vi "4110_Volt _Chan Config Dialog_RTM.vi"(8 "error in (no error)":errorcluster, 11 "CD PTR":T1 format="%.0x") -> (0 "error out":errorcluster, 1 "Channels to Add":u16[](array[numeric]), 2 "Current Limit (out)":dbl, 3 "Initial Voltage Value (out)":dbl, 5 "Cancel (out)":bool)   [LabVIEW 2018, in "NI PXI-4110 Programmable Power Supply Custom Device.lvlib"]
uses:
  NI PXI-4110 Programmable Power Supply Custom Device.lvlib
  <vilib>/NI Veristand/Custom Device API/Custom Device Item Ref.ctl
  Power_Supply_In_Use.ctl
  4110_Global.vi
  <vilib>/NI Veristand/Custom Device API/Get Item Property (U16).vi
  <vilib>/NI Veristand/Custom Device API/Get Item Property (Boolean).vi
  <vilib>/NI VeriStand/Custom Device API/Custom Device API.lvlib
panel:
  in  "Channel(s) to add":T2
  in  "Cancel":bool
  in  "OK Button":bool
  in  "Current Limit":dbl format="%.4f"
  in  "Initial Voltage Value":dbl
  # "Voltage Channels"
  # "Note: Channel 2 current\nvalues will be converted\nto negative values\nappropriately."
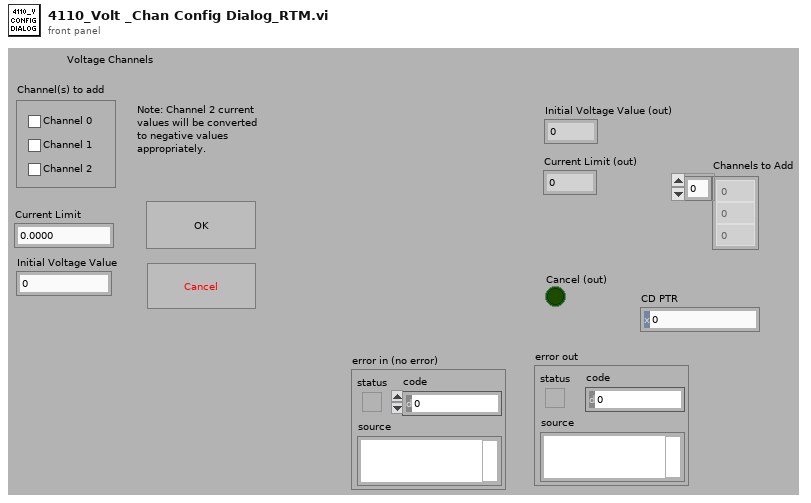
[diagram p1: front panel]
types:
  T1 = typedef "Custom Device API.lvlib/Custom Device Item Ref.ctl" = u64
  T2 = cluster{"Channel 0":bool, "Channel 1":bool, "Channel 2":bool}
  T3 = enum8{"Enabled", "Disabled", "Disabled and Grayed Out"}
  T4 = typedef "NI PXI-4110 Programmable Power Supply Custom Device.lvlib/Power_Supply_In_Use.ctl" = enum16{"PXIe-4112", "PXI-4110"}
  T5 = cluster{"V_min":dbl, "V_max":dbl, "I_min":dbl, "I_max":dbl}
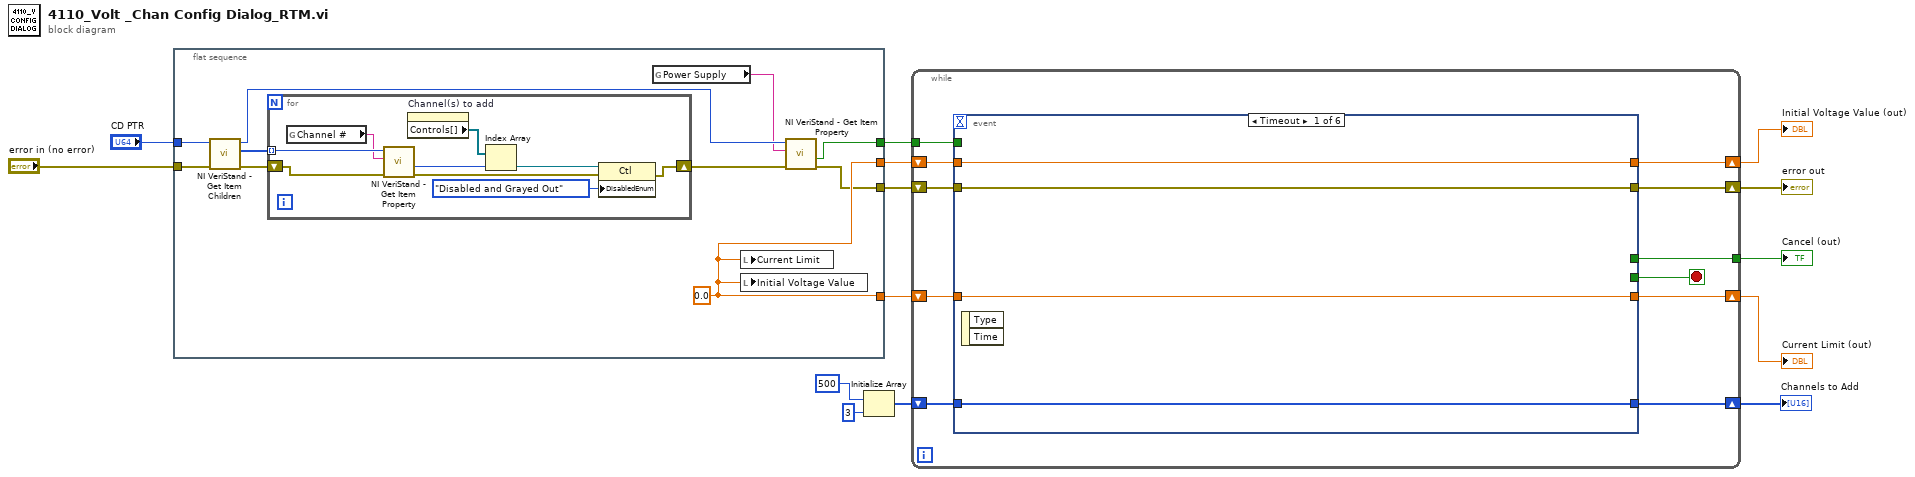
[diagram p0: block diagram]
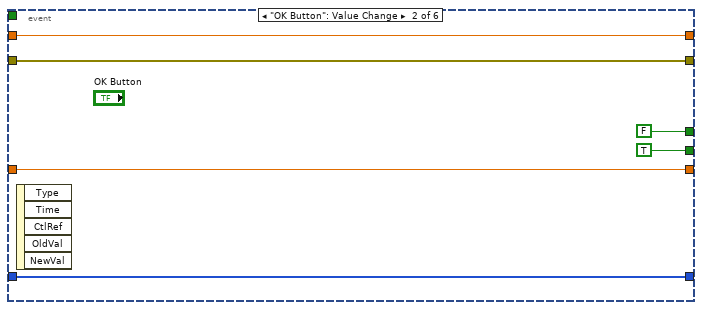
[diagram p2: hidden frame]
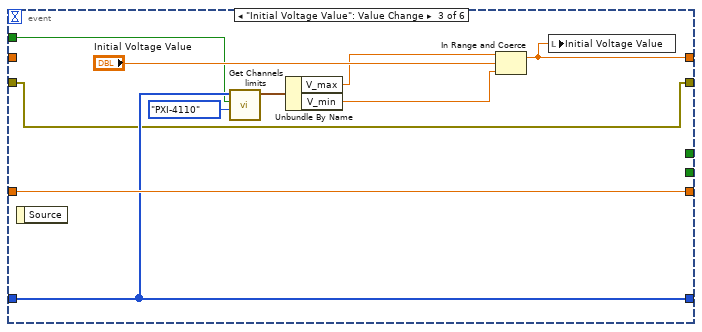
[diagram p3: hidden frame]
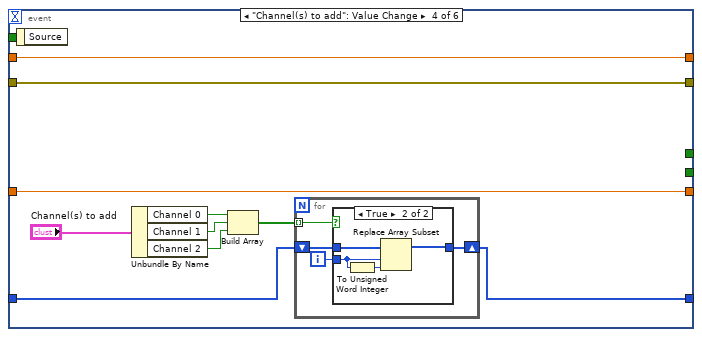
[diagram p4: hidden frame]
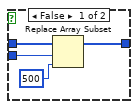
[diagram p5: hidden frame]
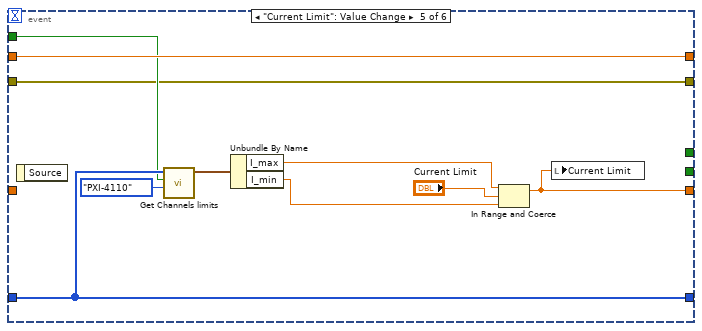
[diagram p6: hidden frame]
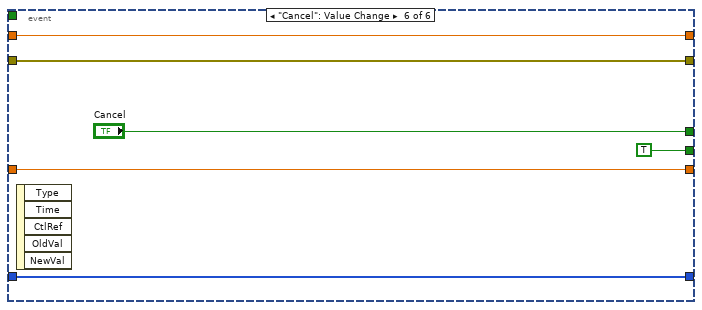
[diagram p7: hidden frame]
diagram:
  n1 = flat-sequence {
    tunnel: [w15] -> w14
    tunnel: [w20] -> w9
    tunnel: [w20] -> w8
    tunnel: "error in (no error)" -> [w24]
    tunnel: "CD PTR" -> [w23]
    tunnel: [w16] -> w5
    frame #0 {
      w20 = 0.0
      n2 = call <vilib>:"NI VeriStand - Get Item Children.vi"("error in (no error)"=w24, "Item Ref in"=w23) -> ("error out"=w21:errorcluster, "Child Refs"=w22:T1[], "Item Ref out"=w18:T1)  [unwired: 6 in, 1 out]
      n3 = for {
        tunnel: w22 -> [w33] mode=indexing
        shift-right: [w25] -> w19
        shift-left: w21 -> [w32]
        n4 = global read "4110_Global.vi" "Channel #"() -> (w31:string)
        n5 = call-poly <vilib>:"NI VeriStand - Get Item Property.vi"("error in (no error)"=w32, "Property Name"=w31, "Item Ref in"=w33) -> ("error out"=w26:errorcluster, "Value"=w27:u16)  [unwired: 5 in, 2 out]
        n6 = property on="Channel(s) to add" class="Clust (strict)"() -> ("Controls[]"=w29:refnum<vi>[])  [unwired: 2 in, 2 out]
        n7 = Index Array(array=w29, index=w27) -> (element=w30:refnum<vi>)
        n8 = property class="Ctl"(reference=w30, error in=w26, "DisabledEnum"=T3."Disabled and Grayed Out" ("Disabled")) -> (error out=w25:errorcluster)  [unwired: 1 out]
      }
      n9 = global read "4110_Global.vi" "Power Supply"() -> (w17:string)
      n10 = local write "Current Limit"(w20) -> ()
      n11 = local write "Initial Voltage Value"(w20) -> ()
      n12 = call-poly <vilib>:"NI VeriStand - Get Item Property.vi"("error in (no error)"=w19, "Property Name"=w17, "Item Ref in"=w18) -> ("error out"=w15:errorcluster, "Value"=w16:bool)  [unwired: 5 in, 2 out]
    }
  }
  n13 = Initialize Array(u16 500 ("element"), 3 ("dimension size")) -> (w2:u16[])
  n14 = while {
    tunnel: [w40] -> w10
    shift-right: [w43] -> w13
    shift-left: w14 -> [w44]
    shift-right: [w42] -> w12
    shift-left: w9 -> [w38]
    shift-right: [w41] -> w11
    shift-left: w8 -> [w37]
    tunnel: w5 -> [w36]
    shift-right: [w34] -> w1
    shift-left: w2 -> [w35]
    stop <- w39 stop-if-true
    n15 = event shown="[0] Timeout" {
      selector: _ -> [_ _ _ _ _ _]
      dyn-events: _ -> [_ _ _ _ _ _]
      timeout: _ -> [_ _ _ _ _ _]
      tunnel: [w48 w51 w64 w74 w95 w100] -> w42
      tunnel: [w47 w50 w62 w73 w94 w99] -> w41
      tunnel: w44 -> [w45 w54 w55 w65 w87 w97]
      tunnel: [w45 w54 w55 w65 w87 w97] -> w43
      tunnel: [_ FALSE ("Cancel") _ _ _ "Cancel"] -> w40
      tunnel: [_ TRUE ("Cancel") _ _ _ TRUE ("Cancel")] -> w39
      tunnel: w38 -> [w48 w51 w64 w74 _ w100]
      tunnel: w37 -> [w47 w50 _ w73 w94 w99]
      tunnel: w36 -> [_ _ w60 _ w92 _]
      tunnel: w35 -> [w46 w49 w61 w67 w93 w98]
      tunnel: [w46 w49 w61 w66 w93 w98] -> w34
      event Timeout {
        n16 = event-data() -> ()  [unwired: 1 in, 2 out]
      }
      event "OK Button": Value Change {
        n17 = event-data() -> ()  [unwired: 1 in, 5 out]
      }
      event "Initial Voltage Value": Value Change {
        n18 = event-data() -> ()  [unwired: 1 in, 1 out]
        n19 = call "Get Channels limits.vi"("Power Supply In Use"=Power_Supply_In_Use."PXI-4110", "External Supply?"=w60, "Channels"=w61) -> ("output cluster"=w58:T5)  [unwired: 7 in, 1 out]
        n20 = Unbundle By Name(w58) -> ("V_max"=w57:dbl, "V_min"=w56:dbl)
        n21 = In Range and Coerce(upper limit=w57, x="Initial Voltage Value", lower limit=w56) -> (coerced(x)=w62:dbl)  [unwired: 1 out]
        n22 = local write "Initial Voltage Value"(w62) -> ()
      }
      event "Channel(s) to add": Value Change {
        n23 = event-data() -> ()  [unwired: 1 in, 1 out]
        n24 = Unbundle By Name("Channel(s) to add") -> ("Channel 0"=w71:bool, "Channel 1"=w70:bool, "Channel 2"=w69:bool)
        n25 = Build Array(w71, w70, w69) -> (w68:bool[])
        n26 = for {
          tunnel: w68 -> [w78] mode=indexing
          shift-right: [w75] -> w66
          shift-left: w67 -> [w77]
          i -> [w76]
          n27 = case shown="True" w78 {
            tunnel: w77 -> [w81 w86]
            tunnel: w76 -> [w82 w84]
            tunnel: [w79 w85] -> w75
            frame False {
              n28 = Replace Array Subset(array=w81, new element=u16 500 ("new element/subarray"), index=w82) -> (w79:u16[])
            }
            frame True {
              n29 = To Unsigned Word Integer(number=w84) -> (unsigned 16bit integer=w83:u16)
              n30 = Replace Array Subset(array=w86, new element=w83, index=w84) -> (w85:u16[])
            }
          }
        }
      }
      event "Current Limit": Value Change {
        n31 = event-data() -> ()  [unwired: 1 in, 1 out]
        n32 = call "Get Channels limits.vi"("Power Supply In Use"=Power_Supply_In_Use."PXI-4110", "External Supply?"=w92, "Channels"=w93) -> ("output cluster"=w90:T5)  [unwired: 7 in, 1 out]
        n33 = Unbundle By Name(w90) -> ("I_max"=w89:dbl, "I_min"=w88:dbl)
        n34 = In Range and Coerce(upper limit=w89, x="Current Limit", lower limit=w88) -> (coerced(x)=w95:dbl)  [unwired: 1 out]
        n35 = local write "Current Limit"(w95) -> ()
      }
      event "Cancel": Value Change {
        n36 = event-data() -> ()  [unwired: 1 in, 5 out]
      }
    }
  }
  "error out" <- w13
  "Current Limit (out)" <- w12
  "Initial Voltage Value (out)" <- w11
  "Cancel (out)" <- w10
  "Channels to Add" <- w1
